vi "GDSII Prototype.vi"() -> ()   [LabVIEW 2019]
panel:
  in  "Raw Data":string
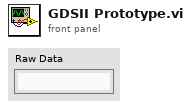
[diagram p1: front panel]
types:
  T1 = enum32{"Invalid", "Standard", "Closed", "Hidden", "Minimized", "Maximized"}
  T2 = enum32{"invalid app kind", "Development System", "Run Time System", "Student Edition", "Embedded LabVIEW", "Evaluation", "Custom"}
  T3 = cluster{"Core":cluster{"Current VI Reference":refnum<vi>, "Close Panel on Exit?":bool}, "Raw Data":string, "Your string data":string}
  T4 = cluster{"Current VI Reference":refnum<vi>, "Close Panel on Exit?":bool}
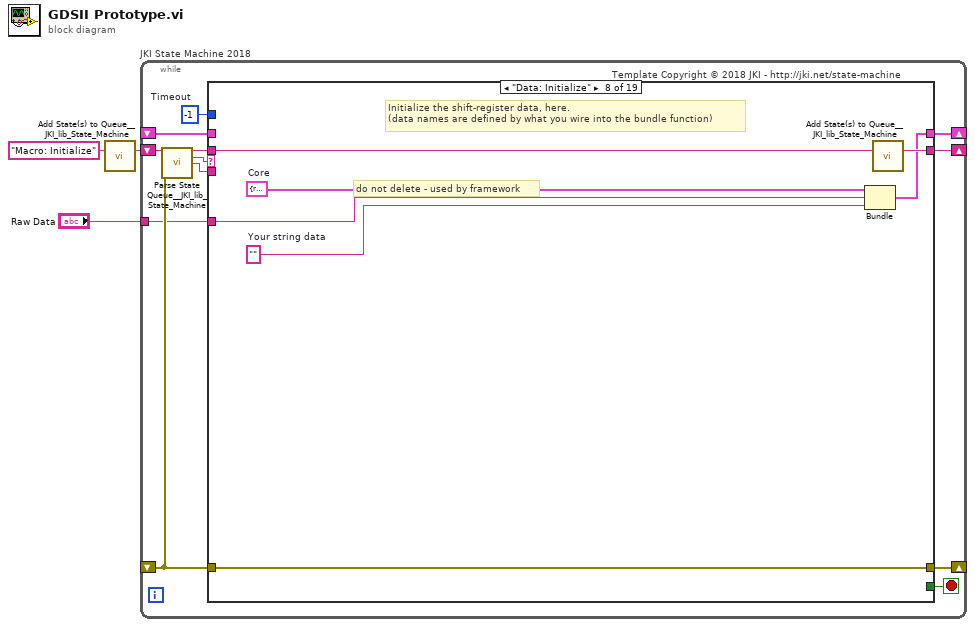
[diagram p0: block diagram]
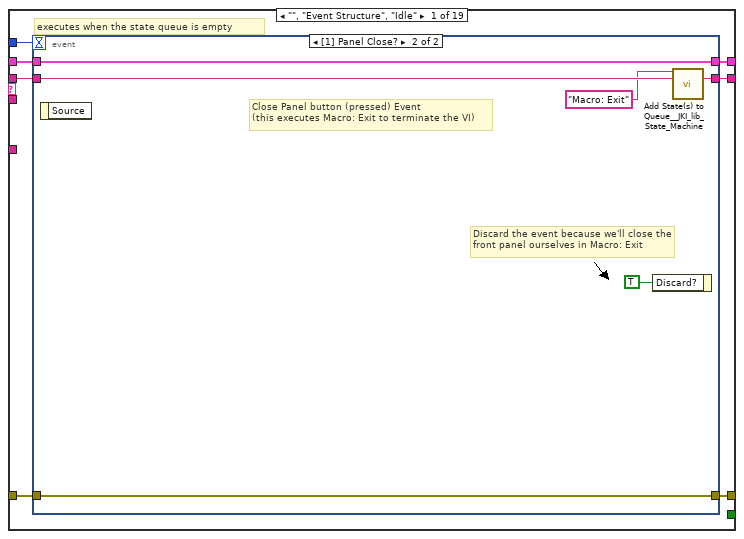
[diagram p2: hidden frame]
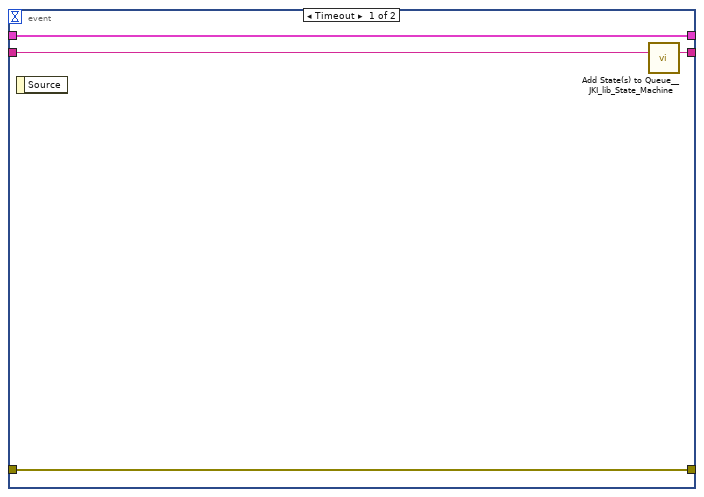
[diagram p3: hidden frame]
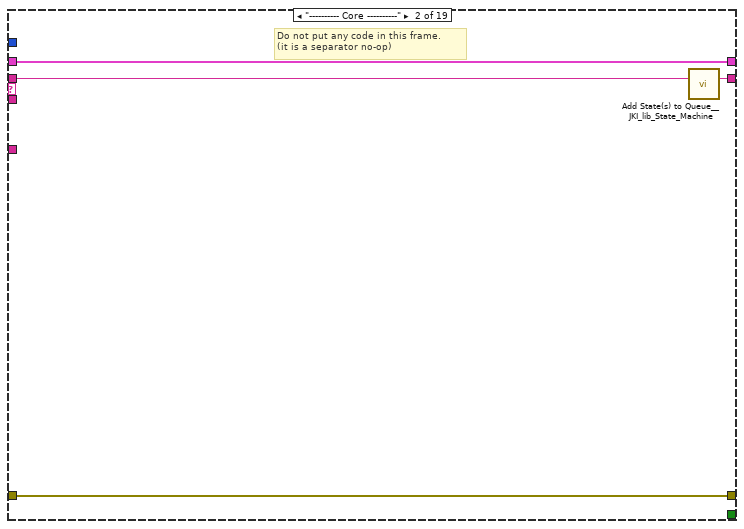
[diagram p4: hidden frame]
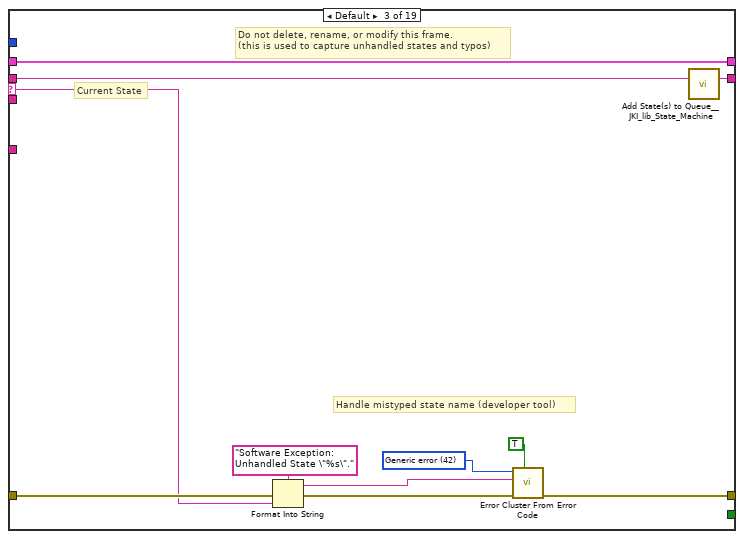
[diagram p5: hidden frame]
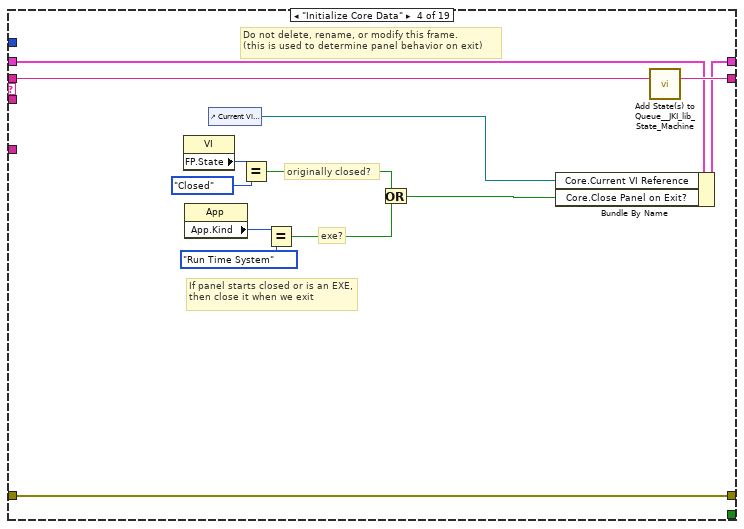
[diagram p6: hidden frame]
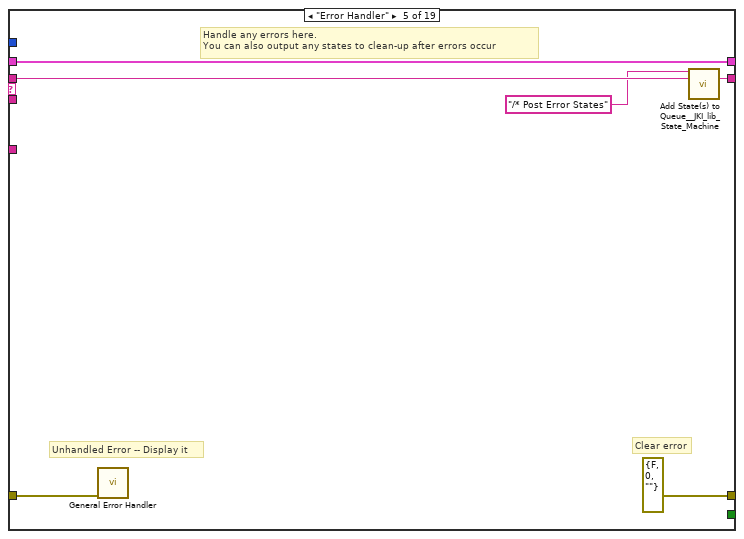
[diagram p7: hidden frame]
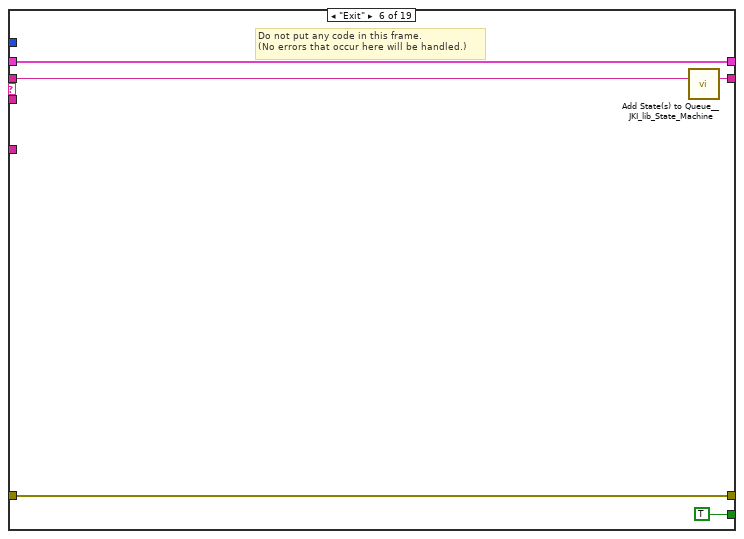
[diagram p8: hidden frame]
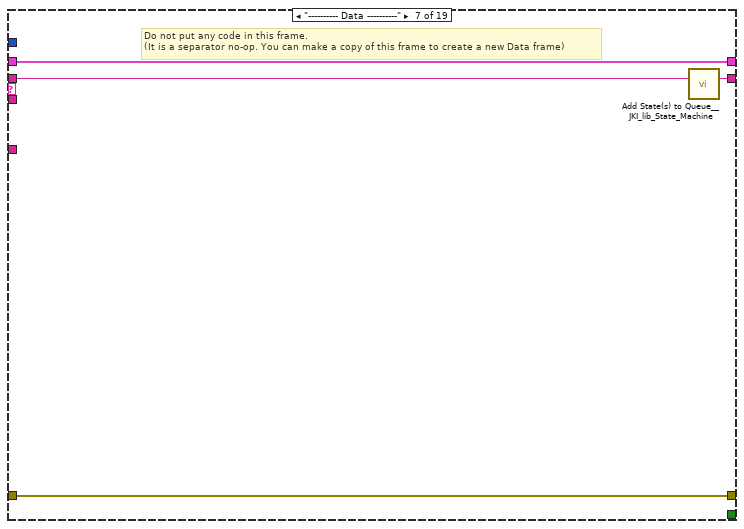
[diagram p9: hidden frame]
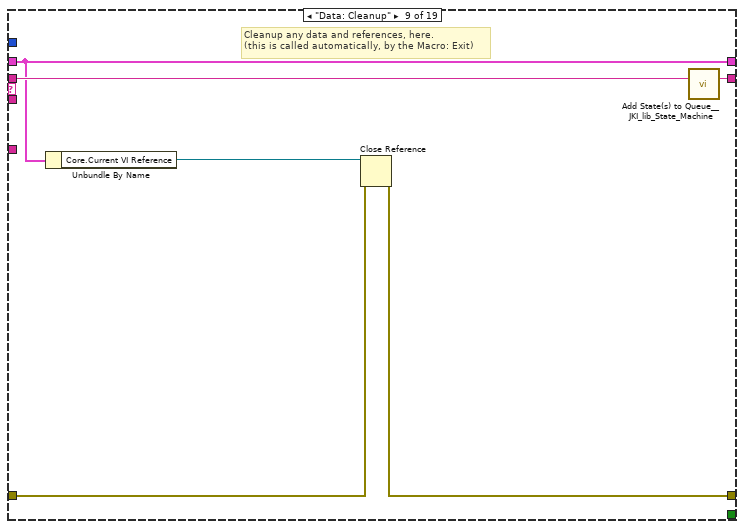
[diagram p10: hidden frame]
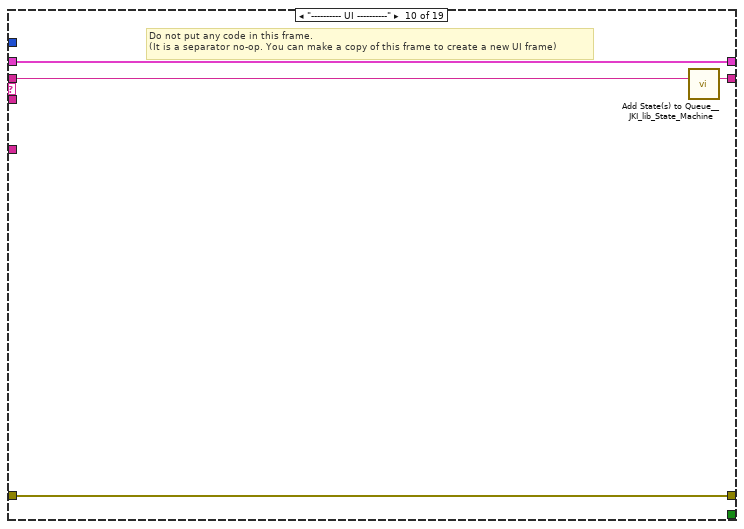
[diagram p11: hidden frame]
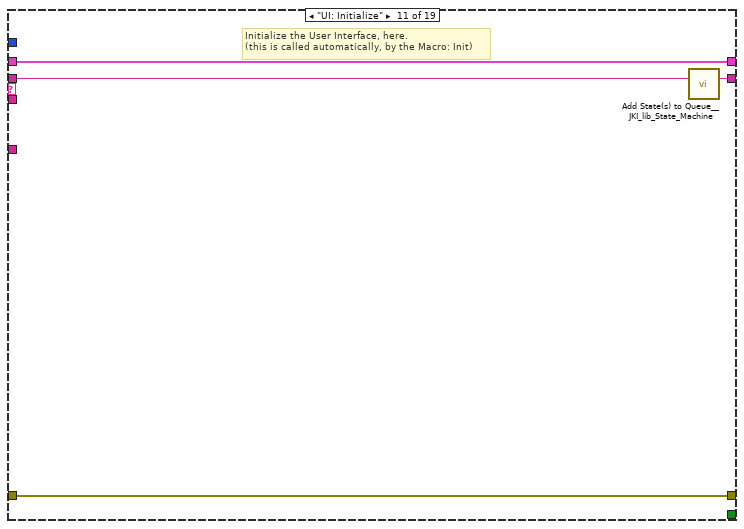
[diagram p12: hidden frame]
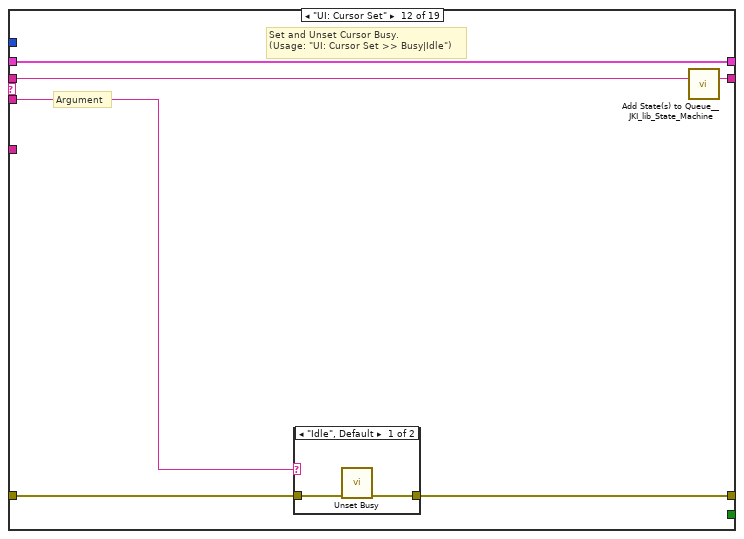
[diagram p13: hidden frame]
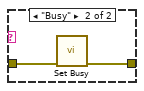
[diagram p14: hidden frame]
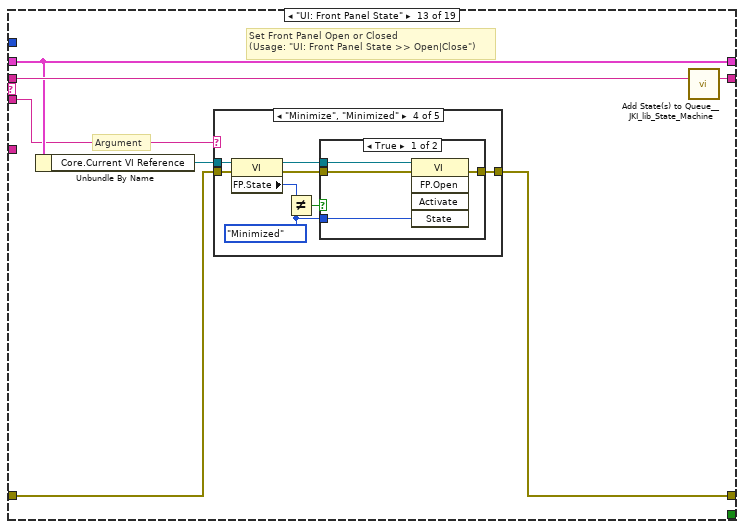
[diagram p15: hidden frame]
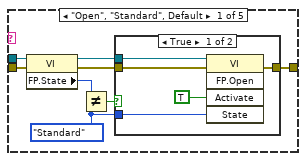
[diagram p16: hidden frame]
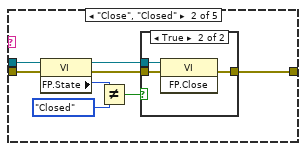
[diagram p18: hidden frame]
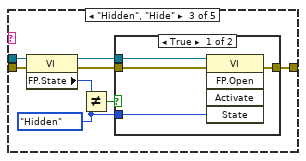
[diagram p20: hidden frame]
diagram:
  n1 = call <vilib>:"Add State(s) to Queue__JKI_lib_State_Machine.vi"("State(s) in (\"\")"="Macro: Initialize") -> ("States Out"=w3:string)  [unwired: 14 in]
  n2 = while "JKI State Machine 2018" {
    shift-right: [w8] -> _
    shift-left: _ -> [w7]
    shift-right: [w11] -> _
    shift-left: _ -> [w5]
    shift-right: [w10] -> _
    shift-left: w3 -> [w12]
    tunnel: "Raw Data" -> [w4]
    stop <- w9 stop-if-true
    w6 = -1  # Timeout
    # "Template Copyright © 2018 JKI - http://jki.net/state-machine"
    n3 = call <vilib>:"Parse State Queue__JKI_lib_State_Machine.vi"("State Queue"=w12, "Error In (no error)"=w5) -> ("Remaining States"=w14:string, "Current State"=w15:string, "Arguments"=w13:string)  [unwired: 11 in]
    n4 = case shown="\"Data: Initialize\"" w15 {
      selector: w15 -> [_ _ w37 _ _ _ _ _ _ _ _ _ _ _ _ _ _ _ _]
      tunnel: w14 -> [w22 w36 w41 w60 w66 w71 w75 w82 w88 w92 w96 w102 w113 w182 w187 w197 w201 w205 w209]
      tunnel: w13 -> [_ _ _ _ _ _ _ _ _ _ _ w97 w107 _ _ _ _ _ _]
      tunnel: w7 -> [w20 w33 w39 w53 w63 w69 w72 _ w83 w89 w94 w100 w109 w179 w184 w194 w198 w202 w206]
      tunnel: [w19 w34 w43 w57 errorcluster {"status"=FALSE, "code"=0, "source"=""} ("error out") w68 w73 w79 w84 w90 w93 w98 w110 w180 w185 w195 w199 w203 w207] -> w11
      tunnel: w5 -> [w18 w34 w42 w57 w62 w68 w73 w79 w85 w90 w93 w99 w111 w180 w185 w195 w199 w203 w207]
      tunnel: [w21 w35 w40 w59 w65 w70 w74 w81 w87 w91 w95 w101 w112 w181 w186 w196 w200 w204 w208] -> w10
      tunnel: [_ _ _ _ _ TRUE _ _ _ _ _ _ _ _ _ _ _ _ _] -> w9
      tunnel: [w17 w33 w39 w58 w63 w69 w72 w80 w83 w89 w94 w100 w109 w179 w184 w194 w198 w202 w206] -> w8
      tunnel: w6 -> [w16 _ _ _ _ _ _ _ _ _ _ _ _ _ _ _ _ _ _]
      tunnel: w4 -> [_ _ _ _ _ _ _ w76 _ _ _ _ _ _ _ _ _ _ _]
      frame "", "Event Structure", "Idle" {
        # "executes when the state queue is empty"
        n5 = event shown="[1] Panel Close?" {
          selector: _ -> [_ _]
          dyn-events: _ -> [_ _]
          timeout: w16 -> [_ _]
          tunnel: w22 -> [w26 w32]
          tunnel: [w25 w31] -> w21
          tunnel: w20 -> [w23 w29]
          tunnel: [w24 w30] -> w19
          tunnel: w18 -> [w24 w30]
          tunnel: [w23 w29] -> w17
          event Timeout {
            n6 = event-data() -> ()  [unwired: 1 in, 1 out]
            n7 = call <vilib>:"Add State(s) to Queue__JKI_lib_State_Machine.vi"("State(s) in (\"\")"=w26) -> ("States Out"=w25:string)  [unwired: 14 in]
          }
          event Panel Close? {
            # "Discard the event because we'll close the front panel ourselves in Macro: Exit"
            # "Close Panel button (pressed) Event\n(this executes Macro: Exit to terminate the VI)"
            n8 = event-data() -> ()  [unwired: 1 in, 1 out]
            n9 = event-data("Discard?"=TRUE) -> ()  [unwired: 1 in, 1 out]
            n10 = call <vilib>:"Add State(s) to Queue__JKI_lib_State_Machine.vi"("State(s) in Front (\"\")"="Macro: Exit", "State(s) in (\"\")"=w32) -> ("States Out"=w31:string)  [unwired: 13 in]
          }
        }
      }
      frame "---------- Core ----------" {
        # "Do not put any code in this frame.\n(it is a separator no-op)"
        n11 = call <vilib>:"Add State(s) to Queue__JKI_lib_State_Machine.vi"("State(s) in (\"\")"=w36) -> ("States Out"=w35:string)  [unwired: 14 in]
      }
      frame Default {
        w46 = 42 items=["No error", "Argument error", "Memory is full", "Out of zone", "End of file", "File already open", "Generic file I/O error", "File not found", "File permission error", "Disk is full", "Duplicate path", "Too many files open", "System feature not enabled", "Resource file not found", "Cannot add resource", "Resource not found", "Image not found", "Image memory error", "Pen does not exist", "Config type invalid", "Config token not found", "Config parse error", "Config memory error", "Bad external code format", "Bad external code offset", "External code not present", "Null window", "Destroy window error", "Null menu", "Print aborted", "Bad print record", "Print driver error", "Windows error during printing", "Memory error during printing", "Print dialog error", "Generic print error", "Invalid device refnum", "Device not found", "Device parameter error", "Device unit error", "Cannot open device", "Device call aborted", "Generic error", "Cancelled by user", "Object ID too low", "Object ID too high", "Object not in heap", "Unknown heap", "Unknown object (invalid DefProc)", "Unknown object (DefProc not in table)", "Message out of range", "Invalid (null) method", "Unknown message", "Manager call not supported", "Bad address", "Network operation in progress", "Network operation timed out", "Connection is busy", "Network attribute not supported", "Network error", "Address in use", "System out of memory", "Connection aborted", "Connection refused", "Not connected", "Already connected", "Connection closed", "Initialization error (interapplication manager)", "Bad occurrence", "Wait on unbound occurrence handler", "Occurrence queue overflow", "Datalog type conflict", "Unused", "Unrecognized type (interapplication manager)", "Memory corrupt", "Failed to make temporary DLL", "Old CIN version", "Drag socket not found", "Failed to load drop-object", "Failed to register OLE object", "Failed to release OLE object", "Format specifier type mismatch", "Unknown format specifier", "Too few format specifiers", "Too many format specifiers", "Scan failed", "Newer CIN version", "Error converting to variant", "Runtime menu error", "Password tampered", "Variant attribute not found", "Incompatible variant data type", "Event data is not available", "Event Store is not present", "Occurrence is not found", "Event Queue is not created", "Event info is not available", "Refnum passed is NULL", "Error retrieving Class GUID", "Error retrieving CoClass GUID", "Error retrieving TypeLib GUID.", "Bad built application magic bytes.", "Specific driver is different from the specific driver associated with the Logical Name.", "There is no session opened to the class driver.", "Max Error", "MAX - Error with config objects", "MAX - Error loading configuration", "MAX - Group not supported"]
        # "Current State"
        # "Do not delete, rename, or modify this frame.\n(this is used to capture unhandled states and typos)"
        # "Handle mistyped state name (developer tool)"
        n12 = Format Into String(format string="Software Exception: Unhandled State \"%s\"." ("message"), error in=w42, w37) -> (resulting string=w45:string, error out=w44:errorcluster)  [unwired: 1 in]
        n13 = call <vilib>:"Error Cluster From Error Code.vi"("show call chain? (False)"=TRUE, "error in (no error)"=w44, "error message (\"\")"=w45, "error code (0)"=w46) -> ("error out"=w43:errorcluster)  [unwired: 5 in]
        n14 = call <vilib>:"Add State(s) to Queue__JKI_lib_State_Machine.vi"("State(s) in (\"\")"=w41) -> ("States Out"=w40:string)  [unwired: 14 in]
      }
      frame "Initialize Core Data" {
        # "Do not delete, rename, or modify this frame.\n(this is used to determine panel behavior on exit)"
        # "originally closed?"
        # "exe?"
        # "If panel starts closed or is an EXE, then close it when we exit"
        n15 = property class="VI"() -> ("FP.State"=w50:T1)  [unwired: 2 in, 2 out]
        n16 = property class="App"() -> ("App.Kind"=w56:T2)  [unwired: 2 in, 2 out]
        n17 = control-ref of="Current VI Reference"() -> (w51:refnum<vi>)
        n18 = Equal?(x=w50, y=T1."Closed" ("Front Panel Window:State")) -> (x = y?=w48:bool)
        n19 = Equal?(x=w56, y=T2."Run Time System" ("Application:Kind")) -> (x = y?=w54:bool)
        n20 = Or(x=w48, y=w54) -> (x .or. y?=w52:bool)
        n21 = Bundle By Name(cluster=w53, "Core.Current VI Reference"=w51, "Core.Close Panel on Exit?"=w52) -> (w58:T3)
        n22 = call <vilib>:"Add State(s) to Queue__JKI_lib_State_Machine.vi"("State(s) in (\"\")"=w60) -> ("States Out"=w59:string)  [unwired: 14 in]
      }
      frame "Error Handler" {
        # "Unhandled Error -- Display it"
        # "Handle any errors here.\nYou can also output any states to clean-up after errors occur"
        # "Clear error"
        n23 = call <vilib>:"General Error Handler.vi"("error in (no error)"=w62) -> ()  [unwired: 10 in, 5 out]
        n24 = call <vilib>:"Add State(s) to Queue__JKI_lib_State_Machine.vi"("State(s) in Front (\"\")"="/* Post Error States", "State(s) in (\"\")"=w66) -> ("States Out"=w65:string)  [unwired: 13 in]
      }
      frame "Exit" {
        # "Do not put any code in this frame.\n(No errors that occur here will be handled.)"
        n25 = call <vilib>:"Add State(s) to Queue__JKI_lib_State_Machine.vi"("State(s) in (\"\")"=w71) -> ("States Out"=w70:string)  [unwired: 14 in]
      }
      frame "---------- Data ----------" {
        # "Do not put any code in this frame.\n(It is a separator no-op. You can make a copy of this frame to create a new Data frame)"
        n26 = call <vilib>:"Add State(s) to Queue__JKI_lib_State_Machine.vi"("State(s) in (\"\")"=w75) -> ("States Out"=w74:string)  [unwired: 14 in]
      }
      frame "Data: Initialize" {
        w78 = T4 {"Current VI Reference"=refnum, "Close Panel on Exit?"=FALSE}  # Core
        w77 = ""  # Your string data
        # "do not delete - used by framework"
        # "Initialize the shift-register data, here.\n(data names are defined by what you wire into the bundle function)"
        n27 = Bundle("Core"=w78, "Raw Data"=w76, "Your string data"=w77) -> (w80:T3)  [unwired: 1 in]
        n28 = call <vilib>:"Add State(s) to Queue__JKI_lib_State_Machine.vi"("State(s) in (\"\")"=w82) -> ("States Out"=w81:string)  [unwired: 14 in]
      }
      frame "Data: Cleanup" {
        # "Cleanup any data and references, here.\n(this is called automatically, by the Macro: Exit)"
        n29 = Unbundle By Name(w83) -> ("Core.Current VI Reference"=w86:refnum<vi>)
        n30 = Close Reference(reference=w86, error in (no error)=w85) -> (error out=w84:errorcluster)
        n31 = call <vilib>:"Add State(s) to Queue__JKI_lib_State_Machine.vi"("State(s) in (\"\")"=w88) -> ("States Out"=w87:string)  [unwired: 14 in]
      }
      frame "---------- UI ----------" {
        # "Do not put any code in this frame.\n(It is a separator no-op. You can make a copy of this frame to create a new UI frame)"
        n32 = call <vilib>:"Add State(s) to Queue__JKI_lib_State_Machine.vi"("State(s) in (\"\")"=w92) -> ("States Out"=w91:string)  [unwired: 14 in]
      }
      frame "UI: Initialize" {
        # "Initialize the User Interface, here.\n(this is called automatically, by the Macro: Init)"
        n33 = call <vilib>:"Add State(s) to Queue__JKI_lib_State_Machine.vi"("State(s) in (\"\")"=w96) -> ("States Out"=w95:string)  [unwired: 14 in]
      }
      frame "UI: Cursor Set" {
        # "Argument"
        # "Set and Unset Cursor Busy.\n(Usage: \"UI: Cursor Set >> Busy|Idle\")"
        n34 = case shown="\"Idle\", Default" w97 {
          tunnel: w99 -> [w104 w106]
          tunnel: [w103 w105] -> w98
          frame "Idle", Default {
            n35 = call <vilib>:"Unset Busy.vi"("error in (no error)"=w104) -> ("error out"=w103:errorcluster)  [unwired: 10 in]
          }
          frame "Busy" {
            n36 = call <vilib>:"Set Busy.vi"("error in (no error)"=w106) -> ("error out"=w105:errorcluster)  [unwired: 9 in, 1 out]
          }
        }
        n37 = call <vilib>:"Add State(s) to Queue__JKI_lib_State_Machine.vi"("State(s) in (\"\")"=w102) -> ("States Out"=w101:string)  [unwired: 14 in]
      }
      frame "UI: Front Panel State" {
        # "Argument"
        # "Set Front Panel Open or Closed\n(Usage: \"UI: Front Panel State >> Open|Close\")"
        n38 = Unbundle By Name(w109) -> ("Core.Current VI Reference"=w108:refnum<vi>)
        n39 = case shown="\"Minimize\", \"Minimized\"" w107 {
          tunnel: w111 -> [w119 w134 w145 w158 w171]
          tunnel: [w121 w135 w147 w160 w173] -> w110
          tunnel: w108 -> [w120 w132 w146 w159 w172]
          frame "Open", "Standard", Default {
            w114 = T1."Standard" ("State")
            n40 = property class="VI"(reference=w120, error in=w119) -> (reference out=w117:refnum<vi>, error out=w118:errorcluster, "FP.State"=w116:T1)
            n41 = Not Equal?(x=w116, y=w114) -> (x != y?=w115:bool)
            n42 = case shown="True" w115 {
              tunnel: [w125 w127] -> w121
              tunnel: w118 -> [w124 w127]
              tunnel: w117 -> [w123 _]
              tunnel: w114 -> [w122 _]
              frame True {
                n43 = invoke class="VI" method="FP.Open"(reference=w123, error in=w124, "Activate"=TRUE, "State"=w122) -> (error out=w125:errorcluster)  [unwired: 1 in, 4 out]
              }
              frame False {
              }
            }
          }
          frame "Close", "Closed" {
            n44 = property class="VI"(reference=w132, error in=w134) -> (reference out=w131:refnum<vi>, error out=w133:errorcluster, "FP.State"=w129:T1)
            n45 = Not Equal?(x=w129, y=T1."Closed" ("Front Panel Window:State")) -> (x != y?=w128:bool)
            n46 = case shown="True" w128 {
              tunnel: [w136 w139] -> w135
              tunnel: w133 -> [w136 w138]
              tunnel: w131 -> [_ w137]
              frame False {
              }
              frame True {
                n47 = invoke class="VI" method="FP.Close"(reference=w137, error in=w138) -> (error out=w139:errorcluster)  [unwired: 1 in, 2 out]
              }
            }
          }
          frame "Hidden", "Hide" {
            w140 = T1."Hidden" ("State")
            n48 = property class="VI"(reference=w146, error in=w145) -> (reference out=w143:refnum<vi>, error out=w144:errorcluster, "FP.State"=w142:T1)
            n49 = Not Equal?(x=w142, y=w140) -> (x != y?=w141:bool)
            n50 = case shown="True" w141 {
              tunnel: [w151 w152] -> w147
              tunnel: w144 -> [w150 w152]
              tunnel: w143 -> [w149 _]
              tunnel: w140 -> [w148 _]
              frame True {
                n51 = invoke class="VI" method="FP.Open"(reference=w149, error in=w150, "State"=w148) -> (error out=w151:errorcluster)  [unwired: 2 in, 4 out]
              }
              frame False {
              }
            }
          }
          frame "Minimize", "Minimized" {
            w153 = T1."Minimized" ("State")
            n52 = property class="VI"(reference=w159, error in=w158) -> (reference out=w156:refnum<vi>, error out=w157:errorcluster, "FP.State"=w155:T1)
            n53 = Not Equal?(x=w155, y=w153) -> (x != y?=w154:bool)
            n54 = case shown="True" w154 {
              tunnel: [w164 w165] -> w160
              tunnel: w157 -> [w163 w165]
              tunnel: w156 -> [w162 _]
              tunnel: w153 -> [w161 _]
              frame True {
                n55 = invoke class="VI" method="FP.Open"(reference=w162, error in=w163, "State"=w161) -> (error out=w164:errorcluster)  [unwired: 2 in, 4 out]
              }
              frame False {
              }
            }
          }
          frame "Maximize", "Maximized" {
            w166 = T1."Maximized" ("State")
            n56 = property class="VI"(reference=w172, error in=w171) -> (reference out=w169:refnum<vi>, error out=w170:errorcluster, "FP.State"=w168:T1)
            n57 = Not Equal?(x=w168, y=w166) -> (x != y?=w167:bool)
            n58 = case shown="True" w167 {
              tunnel: [w177 w178] -> w173
              tunnel: w170 -> [w176 w178]
              tunnel: w169 -> [w175 _]
              tunnel: w166 -> [w174 _]
              frame True {
                n59 = invoke class="VI" method="FP.Open"(reference=w175, error in=w176, "State"=w174) -> (error out=w177:errorcluster)  [unwired: 2 in, 4 out]
              }
              frame False {
              }
            }
          }
        }
        n60 = call <vilib>:"Add State(s) to Queue__JKI_lib_State_Machine.vi"("State(s) in (\"\")"=w113) -> ("States Out"=w112:string)  [unwired: 14 in]
      }
      frame "---------- Macro ----------" {
        # "Do not put any code in this frame.\n(It is a separator no-op. You can make a copy of this frame to create a new Macro frame)"
        n61 = call <vilib>:"Add State(s) to Queue__JKI_lib_State_Machine.vi"("State(s) in (\"\")"=w182) -> ("States Out"=w181:string)  [unwired: 14 in]
      }
      frame "Macro: Initialize" {
        w183 = "Data: Initialize\nInitialize Core Data\nUI: Initialize\n//UI: Front Panel State >> Open"  # Data: Initialize Initialize Core Data UI: Initialize //UI: Front Panel State >> Open
        # "Initialization Macro\n(This is called once, when the VI starts)"
        n62 = call <vilib>:"Add State(s) to Queue__JKI_lib_State_Machine.vi"("State(s) in Front (\"\")"=w183, "State(s) in (\"\")"=w187) -> ("States Out"=w186:string)  [unwired: 13 in]
      }
      frame "Macro: Exit" {
        # "Exit Macro\n(This is called once, when the VI exits)"
        n63 = Unbundle By Name(w194) -> ("Core.Close Panel on Exit?"=w193:bool)
        n64 = Select(t="UI: Front Panel State >> Close", s=w193, f="") -> (s? t:f=w190:string)
        n65 = call <vilib>:"Add State(s) to Queue__JKI_lib_State_Machine.vi"("State(s) in (\"\")"=w190, "State(s) at Back (\"\")"="Data: Cleanup\nExit") -> ("States Out"=w188:string)  [unwired: 13 in]
        n66 = call <vilib>:"Add State(s) to Queue__JKI_lib_State_Machine.vi"("State(s) in Front (\"\")"=w188, "State(s) in (\"\")"=w197) -> ("States Out"=w196:string)  [unwired: 13 in]
      }
      frame "---------- Header ----------" {
        # "Template Separator\n(You can make a copy of, or modify, this frame)"
        n67 = call <vilib>:"Add State(s) to Queue__JKI_lib_State_Machine.vi"("State(s) in (\"\")"=w201) -> ("States Out"=w200:string)  [unwired: 14 in]
      }
      frame "Header: Record Type" {
        # "Your code here.\n(You can make a copy of, or modify, this frame)"
        n68 = call <vilib>:"Add State(s) to Queue__JKI_lib_State_Machine.vi"("State(s) in (\"\")"=w205) -> ("States Out"=w204:string)  [unwired: 14 in]
      }
      frame "Header: 2" {
        # "Your code here.\n(You can make a copy of, or modify, this frame)"
        n69 = call <vilib>:"Add State(s) to Queue__JKI_lib_State_Machine.vi"("State(s) in (\"\")"=w209) -> ("States Out"=w208:string)  [unwired: 14 in]
      }
    }
  }
